vi "CheckAveragingDEM.vi"(9 "FPGA in":refnum<queue>) -> (2 "Averaging":bool, 3 "FPGA out":refnum<queue>)   [LabVIEW 2019, in "FPGA.lvlib"]
uses:
  FPGA.lvlib
  FPGA.ctl
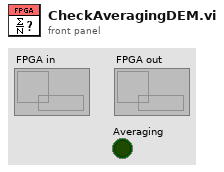
[diagram p1: front panel]
types:
  T1 = typedef "FPGA.lvlib/FPGA.ctl" = cluster{"Start freq. [Hz]":dbl, "Sweep duration [s]":dbl, "Freq. step [Hz]":dbl, "DAC Sample Rate":dbl, "ADC Sample Rate":dbl, "CMD port":u16, "DFAST port":u16, "CMD ID":refnum<k16>, "DFAST ID":refnum<k16>, "CMD error out":errorcluster, "FPGA IP":string, "DFAST error out ":errorcluster, "Stop freq. [Hz]":dbl, "Discrete sweep":bool, "Initial NCO":u32, "Difference NCO":i32, "step NCO":i64, "Final NCO":u32, "clocks for step":u32, "demodulation":bool, "NCO Phase Precision":u32, "NCO Sample Rate":dbl, "Time for step [s]":dbl, "NCO freq. resolution":dbl, "Sweep speed [Hz/s]":dbl, "Connected":bool, "Slew Rate [V/us]":dbl, "Parameters_ok":bool, "Amplitude [mVpp]":dbl, "Scale Factor":fxp<+,16,0>, "Acquiring":bool, "DAC-ADC Latency":u16, "Digital Gain":i32, "Number of steps":i32, "Averaging preferred":bool, "Filter Order":u32, "Settling":enum16{"99%", "99,9%"}}
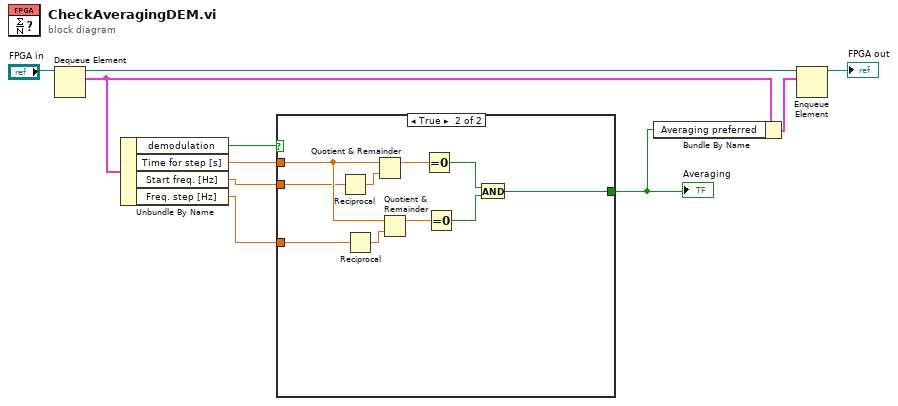
[diagram p0: block diagram]
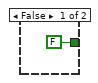
[diagram p2: hidden frame]
diagram:
  n1 = Dequeue Element(queue="FPGA in") -> (queue out=w8:refnum<queue>, element=w3:T1)  [unwired: 2 in, 2 out]
  n2 = Unbundle By Name(w3) -> ("demodulation"=w7:bool, "Time for step [s]"=w6:dbl, "Start freq. [Hz]"=w5:dbl, "Freq. step [Hz]"=w4:dbl)
  n3 = case shown="True" w7 {
    tunnel: w6 -> [_ w19]
    tunnel: w5 -> [_ w18]
    tunnel: w4 -> [_ w17]
    tunnel: [FALSE w12] -> w1
    frame False {
    }
    frame True {
      n4 = Reciprocal(x=w18) -> (1/x=w21:dbl)
      n5 = Reciprocal(x=w17) -> (1/x=w20:dbl)
      n6 = Quotient & Remainder(x=w19, y=w21) -> (x-y*floor(x/y)=w16:dbl)  [unwired: 1 out]
      n7 = Quotient & Remainder(x=w19, y=w20) -> (x-y*floor(x/y)=w15:dbl)  [unwired: 1 out]
      n8 = Equal To 0?(x=w16) -> (x = 0?=w14:bool)
      n9 = Equal To 0?(x=w15) -> (x = 0?=w13:bool)
      n10 = And(x=w14, y=w13) -> (x .and. y?=w12:bool)
    }
  }
  "Averaging" <- w1
  n11 = Bundle By Name(cluster=w3, "Averaging preferred"=w1) -> (w2:T1)
  n12 = Enqueue Element(queue=w8, element=w2) -> (queue out=→"FPGA out":refnum<queue>)  [unwired: 2 in, 2 out]
